vi "gripper_control.vi"(2 "Estado_Gripper":bool, 3 "Estado_Robot":dbl) -> (1 "Angulo_Gripper":dbl)   [LabVIEW 2019]
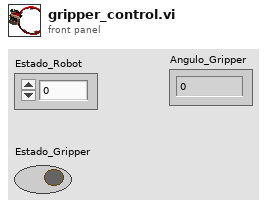
[diagram p1: front panel]
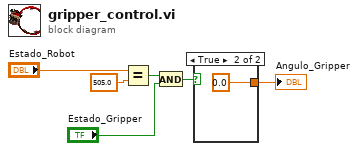
[diagram p0: block diagram]
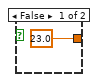
[diagram p2: hidden frame]
diagram:
  n1 = Equal?(x="Estado_Robot", y=505.0) -> (x = y?=w3:bool)
  n2 = And(x=w3, y="Estado_Gripper") -> (x .and. y?=w1:bool)
  n3 = case shown="True" w1 {
    tunnel: [23.0 0.0] -> w6
    frame False {
    }
    frame True {
    }
  }
  "Angulo_Gripper" <- w6
